vi "test change fails and produces message and actual file.vi"(8 "error in (no error)":errorcluster, 11 "TestCase in":refnum<class "Testing Approval Tests.lvclass">) -> (0 "error out":errorcluster, 3 "TestCase out":refnum<class "Testing Approval Tests.lvclass">)   [LabVIEW 2020, in "Testing Approval Tests.lvclass"]
uses:
  Testing Approval Tests.lvclass
  <vilib>/addons/_JKI Toolkits/VI Tester/TestCase.llb/TestCase.lvclass
  C:/Program Files/National Instruments/LabVIEW 2020/vi.lib/addons/_JKI Toolkits/VI Tester/TestCase.llb/TestCase.lvclass
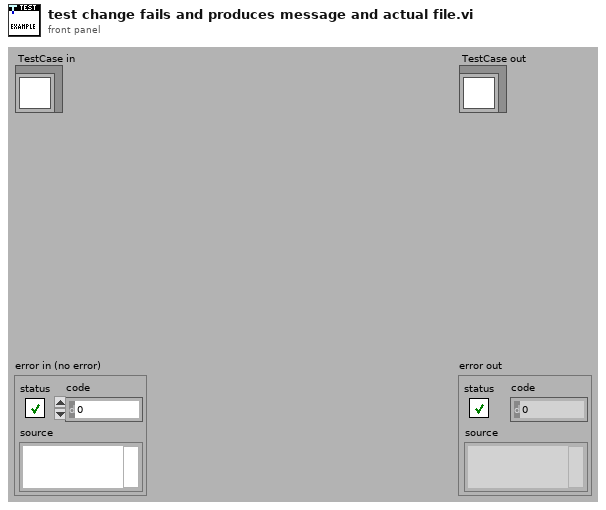
[diagram p1: front panel]
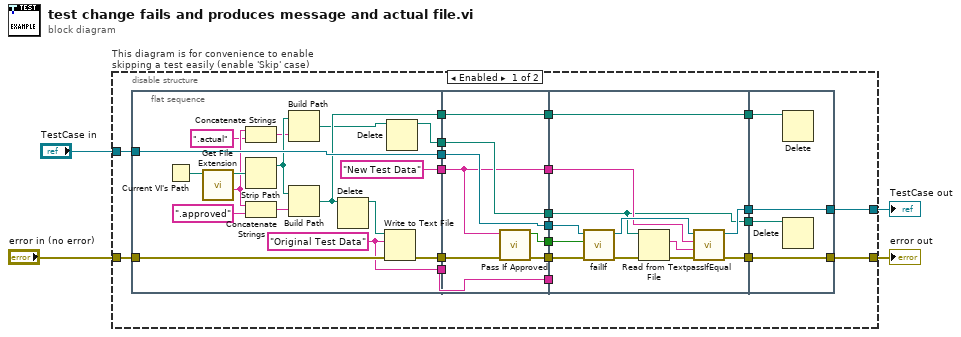
[diagram p0: block diagram]
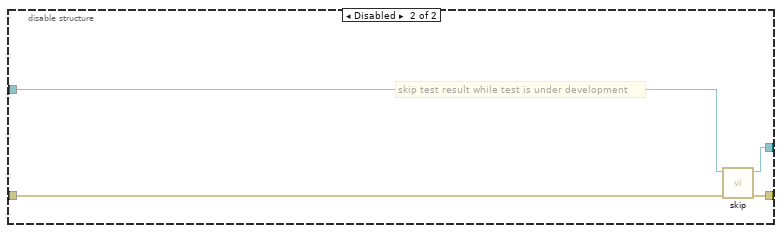
[diagram p2: hidden frame]
diagram:
  n1 = disable-structure "This diagram is for convenience to enable skipping a test easily (enable 'Skip' case)" shown="Enabled" {
    disable-tunnel: "TestCase in" -> [w17 w70]
    disable-tunnel: [w16 w68] -> w1
    disable-tunnel: [w24 w69] -> w3
    disable-tunnel: "error in (no error)" -> [w25 w67]
    frame Enabled {
      n2 = flat-sequence {
        tunnel: w25 -> [w38]
        tunnel: [w37] -> w23
        tunnel: [w42] -> w18
        tunnel: w17 -> [w42]
        tunnel: ["New Test Data"] -> w15
        tunnel: [w35] -> w11
        tunnel: [w27] -> w9
        tunnel: [w26] -> w7
        tunnel: w23 -> [w49]
        tunnel: [w48] -> w22
        tunnel: [w50] -> w19
        tunnel: w18 -> [w50]
        tunnel: w15 -> [w44]
        tunnel: [w47] -> w14
        tunnel: [w46] -> w12
        tunnel: w11 -> [w46]
        tunnel: [w45] -> w10
        tunnel: w9 -> [w45]
        tunnel: [w44] -> w8
        tunnel: w7 -> [w43]
        tunnel: [w43] -> w6
        tunnel: w22 -> [w62]
        tunnel: [w56] -> w21
        tunnel: [w54] -> w20
        tunnel: w19 -> [w60]
        tunnel: w14 -> [w59]
        tunnel: [w58] -> w13
        tunnel: w12 -> [w58]
        tunnel: w10 -> [w51]
        tunnel: w8 -> [w53]
        tunnel: w6 -> [_]
        tunnel: [w51] -> w5
        tunnel: [w66] -> w24
        tunnel: w21 -> [w66]
        tunnel: [w65] -> w16
        tunnel: w20 -> [w65]
        tunnel: w13 -> [w64]
        tunnel: w5 -> [w63]
        frame #0 {
          w26 = "Original Test Data"
          n3 = Current VI's Path() -> (path=w41:path)
          n4 = call <vilib>:"Get File Extension.vi"("file"=w41) -> ("filename without extension"=w32:string, "dup file"=w40:path)  [unwired: 6 in, 3 out]
          n5 = Concatenate Strings(w32, ".actual" ("string")) -> (w28:string)
          n6 = Strip Path(path=w40) -> (stripped path=w29:path)  [unwired: 1 out]
          n7 = Concatenate Strings(w32, ".approved" ("string")) -> (w33:string)
          n8 = Build Path(base path=w29, name or relative path=w28) -> (appended path=w30:path)
          n9 = Build Path(base path=w29, name or relative path=w33) -> (appended path=w35:path)
          n10 = Delete(path (use dialog)=w35) -> (deleted path=w36:path)  [unwired: 4 in, 2 out]
          n11 = Write to Text File(file (use dialog)=w36, text=w26, error in=w38) -> (error out=w37:errorcluster)  [unwired: 1 in, 2 out]
          n12 = Delete(path (use dialog)=w30) -> (deleted path=w27:path)  [unwired: 4 in, 2 out]
        }
        frame #1 {
          n13 = call "Pass If Approved.vi"("error in (no error)"=w49, "Test Data"=w44) -> ("error out"=w48:errorcluster, "Passed?"=w47:bool)  [unwired: 7 in, 1 out]
        }
        frame #2 {
          n14 = call-dynamic "failIf.vi"("error in (no error)"=w62, "fail"=w59, "TestCase in"=w60) -> ("error out"=w61:errorcluster, "TestCase out"=w55:refnum<class "Testing Approval Tests.lvclass">)  [unwired: 7 in]
          n15 = Read from Text File(file (use dialog)=w51, error in=w61) -> (text=w52:string, error out=w57:errorcluster)  [unwired: 2 in, 2 out]
          n16 = call-dynamic "passIfEqual.vi"("error in (no error)"=w57, "y"=w52, "x"=w53, "TestCase in"=w55) -> ("error out"=w56:errorcluster, "TestCase out"=w54:refnum<class "Testing Approval Tests.lvclass">)  [unwired: 6 in]
        }
        frame #3 {
          n17 = Delete(path (use dialog)=w64) -> ()  [unwired: 4 in, 3 out]
          n18 = Delete(path (use dialog)=w63) -> ()  [unwired: 4 in, 3 out]
        }
      }
    }
    frame Disabled {
      # "skip test result while test is under development"
      n19 = call <vilib>:"skip.vi"("error in (no error)"=w67, "TestCase in"=w70) -> ("error out"=w69:errorcluster, "TestCase out"=w68:refnum<class "Testing Approval Tests.lvclass">)  [unwired: 8 in]
    }
  }
  "error out" <- w3
  "TestCase out" <- w1
